vi "cos_rise_512_steps.vi"(9 "new step":bool, 10 "input valid":bool=TRUE, 11 "data in":fxp<+/-,16,1>) -> (1 "output valid":bool, 2 "steping":bool, 3 "data out":fxp<+/-,16,1>)   [LabVIEW 2021]
doc: "rise function.\n32 steps of half cos."
uses:
  <instrlib>/_niInstr/Basic Elements/v1/FPGA/Private/Count Up U16.vi
  <vilib>/rvi/FXPMathLib/FxpSub/XNode/nifxpmath_Sub.xnode
  <vilib>/rvi/FXPMathLib/FxpMul/XNode/nifxpmath_Multiplier.xnode
  <vilib>/rvi/FXPMathLib/FxpAdd/XNode/nifxpmath_Add.xnode
  <instrlib>/_niInstr/Basic Elements/v1/FPGA/niInstr Basic Elements v1 FPGA.lvlib
  <vilib>/rvi/FXPMathLib/sim/FxpSim.dll
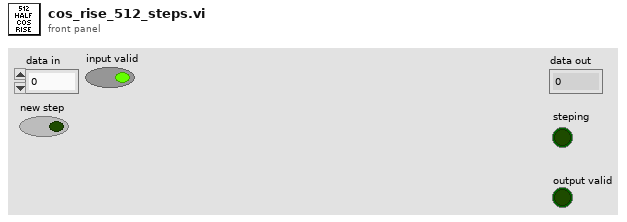
[diagram p1: front panel]
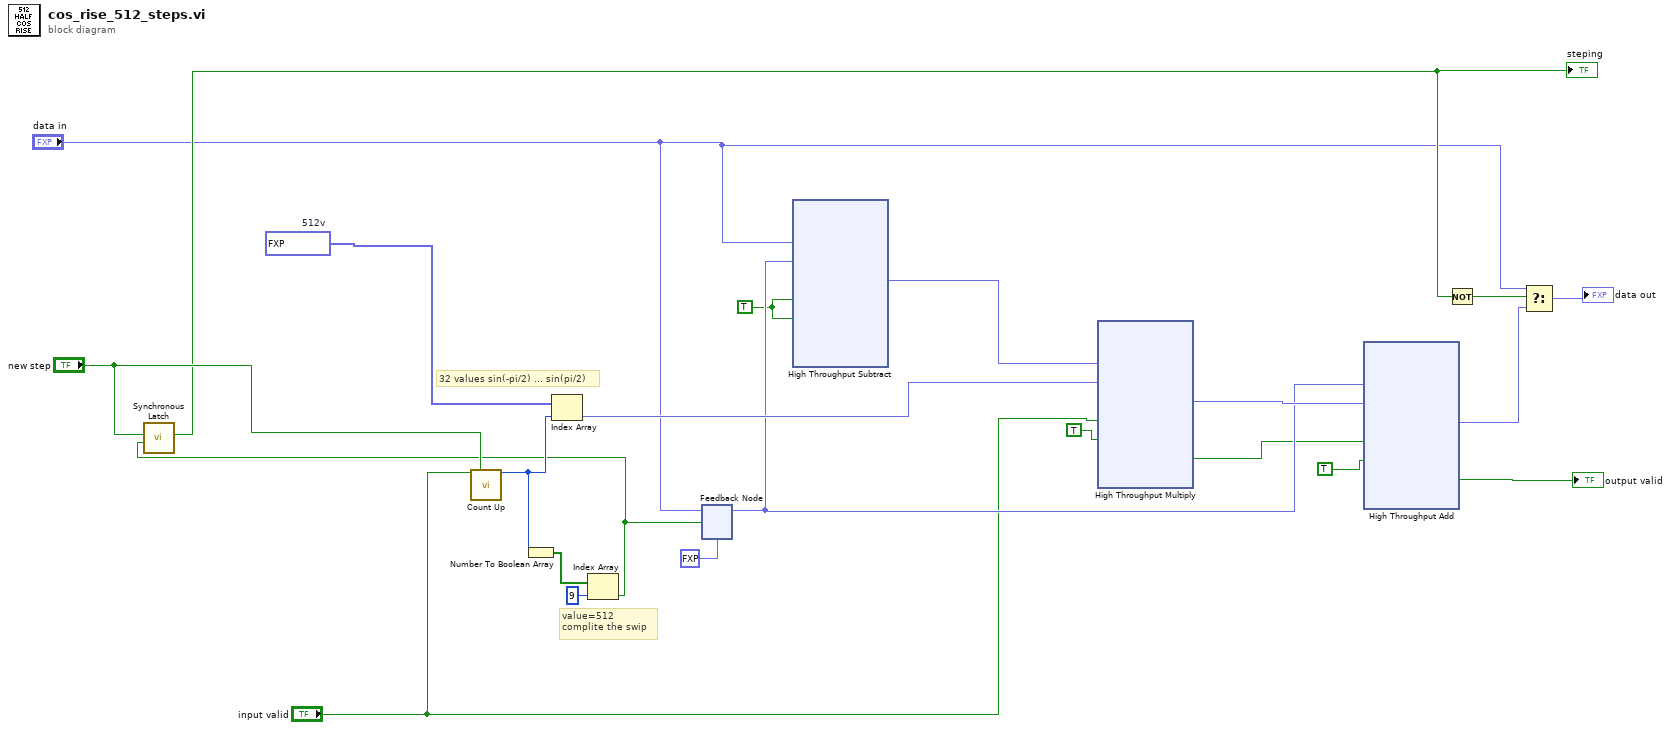
[diagram p0: block diagram]
diagram:
  w5 = fxp<+,24,0>[] [9.417533874511719e-06, 3.7670135498046875e-05, 8.469820022583008e-05, 0.00015056133270263672, 0.0002353191375732422, 0.0003387928009033203, 0.00046116113662719727, 0.0006022453308105469, 0.0007622241973876953, 0.0009409189224243164, 0.001138448715209961, 0.0013547539710998535, 0.0015898346900939941, 0.0018436908721923828, 0.0021163225173950195, 0.0024076104164123535, 0.002717733383178711, 0.0030465126037597656, 0.003394007682800293, 0.003760218620300293, 0.004145145416259766, 0.00454866886138916, 0.004970908164978027, 0.005411744117736816, 0.005871236324310303, 0.0063492655754089355, 0.006845951080322266, 0.007361173629760742, 0.007894933223724365, 0.008447229862213135, 0.00901806354522705, 0.009607374668121338, 0.01021510362625122, 0.010841310024261475, 0.011485934257507324, 0.012148916721343994, 0.01283031702041626, 0.01353001594543457, 0.014248073101043701, 0.014984369277954102, 0.015738964080810547, 0.016511738300323486, 0.017302751541137695, 0.0181119441986084, 0.018939316272735596, 0.019784748554229736, 0.02064824104309082, 0.021529853343963623, 0.02242940664291382, 0.02334696054458618, 0.024282515048980713, 0.025235891342163086, 0.02620720863342285, 0.02719634771347046, 0.028203248977661133, 0.02922797203063965, 0.030270397663116455, 0.03133046627044678, 0.03240823745727539, 0.033503592014312744, 0.03461652994155884, 0.03574693202972412, 0.03689485788345337, 0.03806024789810181, 0.03924298286437988, 0.0404430627822876, 0.04166048765182495, 0.04289513826370239, 0.044146955013275146, 0.04541599750518799, 0.04670214653015137, 0.04800534248352051, 0.04932558536529541, 0.05066275596618652, 0.05201685428619385, 0.05338782072067261, 0.0547756552696228, 0.05618017911911011, 0.0576014518737793, 0.05903935432434082, 0.06049388647079468, 0.06196492910385132, 0.06345248222351074, 0.06495648622512817, 0.06647688150405884, 0.06801354885101318, 0.06956654787063599, 0.07113569974899292, 0.07272100448608398, 0.0743224024772644, 0.0759398341178894, 0.07757323980331421, 0.07922250032424927, 0.08088767528533936, 0.08256858587265015, 0.08426517248153687, 0.08597749471664429, 0.08770537376403809, 0.08944875001907349, 0.09120756387710571, 0.09298181533813477, 0.0947713851928711, 0.09657621383666992, 0.09839624166488647, 0.1002313494682312, 0.1020815372467041, 0.10394668579101562, 0.10582679510116577, 0.10772168636322021, 0.10963135957717896, 0.11155575513839722, 0.11349475383758545, 0.11544835567474365, 0.1174163818359375, 0.11939883232116699, 0.12139558792114258, 0.12340658903121948, 0.12543177604675293, 0.12747108936309814, 0.12952440977096558, 0.13159173727035522, 0.13367289304733276, 0.13576781749725342, 0.1378764510154724, 0.13999873399734497, 0.14213460683822632, 0.14428389072418213, 0.1464465856552124, 0.14862263202667236, 0.15081185102462769, 0.15301424264907837, 0.15522974729537964, 0.15745818614959717, 0.15969949960708618, 0.1619536280632019, 0.16422051191329956, 0.1665000319480896, 0.16879212856292725, 0.17109668254852295, 0.17341357469558716, 0.17574280500411987, 0.17808425426483154, 0.18043780326843262, 0.18280333280563354, 0.1851809024810791, 0.18757027387619019, 0.18997138738632202, 0.19238418340682983, 0.19480860233306885, 0.19724446535110474, 0.1996917724609375, 0.2021503448486328, 0.2046201229095459, 0.20710104703903198, 0.2095929980278015, 0.21209591627120972, 0.21460962295532227, 0.21713411808013916, 0.21966922283172607, 0.22221487760543823, 0.22477102279663086, 0.22733747959136963, 0.22991424798965454, 0.23250120878219604, 0.23509818315505981, 0.23770517110824585, 0.24032199382781982, 0.24294865131378174, 0.2455849051475525, 0.24823081493377686, 0.25088614225387573, 0.2535508871078491, 0.25622493028640747, 0.25890809297561646, 0.2616003751754761, 0.2643016576766968, 0.26701176166534424, 0.2697306275367737, 0.27245819568634033, 0.27519434690475464, 0.2779389023780823, 0.28069186210632324, 0.283453106880188, 0.2862224578857422, 0.28899985551834106, 0.29178524017333984, 0.2945784330368042, 0.2973793148994446, 0.300187885761261, 0.3030039668083191, 0.3058274984359741, 0.30865830183029175, 0.3114963173866272, 0.3143414258956909, 0.31719350814819336, 0.32005250453948975, 0.32291823625564575, 0.3257906436920166, 0.3286696672439575, 0.3315550684928894, 0.33444684743881226, 0.33734482526779175, 0.3402490019798279, 0.34315913915634155, 0.346075177192688, 0.34899699687957764, 0.3519245386123657, 0.3548576831817627, 0.35779625177383423, 0.36074018478393555, 0.3636893033981323, 0.36664360761642456, 0.36960291862487793, 0.37256717681884766, 0.3755362033843994, 0.3785099387168884, 0.38148820400238037, 0.38447093963623047, 0.38745802640914917, 0.3904494047164917, 0.39344483613967896, 0.39644432067871094, 0.3994476795196533, 0.40245485305786133, 0.40546566247940063, 0.40848004817962646, 0.41149789094924927, 0.4145190715789795, 0.4175434112548828, 0.42057090997695923, 0.4236013889312744, 0.4266347885131836, 0.42967087030410767, 0.43270963430404663, 0.43575096130371094, 0.43879467248916626, 0.4418407082557678, 0.4448888897895813, 0.4479391574859619, 0.4509914517402649, 0.45404553413391113, 0.45710134506225586, 0.4601587653160095, 0.46321773529052734, 0.4662780165672302, 0.46933960914611816, 0.4724023938179016, 0.47546619176864624, 0.4785308837890625, 0.4815964102745056, 0.48466259241104126, 0.48772937059402466, 0.49079662561416626, 0.4938642382621765, 0.4969320297241211, 0.5, 0.5030679702758789, 0.5061357617378235, 0.5092033743858337, 0.5122706294059753, 0.5153374075889587, 0.5184035897254944, 0.5214691162109375, 0.5245338082313538, 0.5275976061820984, 0.5306603908538818, 0.5337219834327698, 0.5367822647094727, 0.5398412346839905, 0.5428986549377441, 0.5459544658660889, 0.5490085482597351, 0.5520608425140381, 0.5551111102104187, 0.5581592917442322, 0.5612053275108337, 0.5642490386962891, 0.5672903656959534, 0.5703291296958923, 0.5733652114868164, 0.5763986110687256, 0.5794290900230408, 0.5824565887451172, 0.5854809284210205, 0.5885021090507507, 0.5915199518203735, 0.5945343375205994, 0.5975451469421387, 0.6005523204803467, 0.6035556793212891, 0.606555163860321, 0.6095505952835083, 0.6125419735908508, 0.6155290603637695, 0.6185117959976196, 0.6214900612831116, 0.6244637966156006, 0.6274328231811523, 0.6303970813751221, 0.6333563923835754, 0.6363106966018677, 0.6392598152160645, 0.6422037482261658, 0.6451423168182373, 0.6480754613876343, 0.6510030031204224, 0.653924822807312, 0.6568408608436584, 0.6597509980201721, 0.6626551747322083, 0.6655531525611877, 0.6684449315071106, 0.6713303327560425, 0.6742093563079834, 0.6770817637443542, 0.6799474954605103, 0.6828064918518066, 0.6856585741043091, 0.6885036826133728, 0.6913416981697083, 0.6941725015640259, 0.6969960331916809, 0.699812114238739, 0.7026206851005554, 0.7054215669631958, 0.7082147598266602, 0.7110001444816589, 0.7137775421142578, 0.716546893119812, 0.7193081378936768, 0.7220610976219177, 0.7248056530952454, 0.7275418043136597, 0.7302693724632263, 0.7329882383346558, 0.7356983423233032, 0.7383996248245239, 0.7410919070243835, 0.7437750697135925, 0.7464491128921509, 0.7491138577461243, 0.7517691850662231, 0.7544150948524475, 0.7570513486862183, 0.7596780061721802, 0.7622948288917542, 0.7649018168449402, 0.767498791217804, 0.7700857520103455, 0.7726625204086304, 0.7752289772033691, 0.7777851223945618, 0.7803307771682739, 0.7828658819198608, 0.7853903770446777, 0.7879040837287903, 0.7904070019721985, 0.792898952960968, 0.7953798770904541, 0.7978496551513672, 0.8003082275390625, 0.8027555346488953, 0.8051913976669312, 0.8076158165931702, 0.810028612613678, 0.8124297261238098, 0.8148190975189209, 0.8171966671943665, 0.8195621967315674, 0.8219157457351685, 0.8242571949958801, 0.8265864253044128, 0.828903317451477, 0.8312078714370728, 0.8334999680519104, 0.8357794880867004, 0.8380463719367981, 0.8403005003929138, 0.8425418138504028, 0.8447702527046204, 0.8469857573509216, 0.8491881489753723, 0.8513773679733276, 0.8535534143447876, 0.8557161092758179, 0.8578653931617737, 0.860001266002655, 0.8621235489845276, 0.8642321825027466, 0.8663271069526672, 0.8684082627296448, 0.8704755902290344, 0.8725289106369019, 0.8745682239532471, 0.8765934109687805, 0.8786044120788574, 0.880601167678833, 0.8825836181640625, 0.8845516443252563, 0.8865052461624146, 0.8884442448616028, 0.890368640422821, 0.8922783136367798, 0.8941732048988342, 0.8960533142089844, 0.8979184627532959, 0.8997686505317688, 0.9016037583351135, 0.9034237861633301, 0.9052286148071289, 0.9070181846618652, 0.9087924361228943, 0.9105512499809265, 0.9122946262359619, 0.9140225052833557, 0.9157348275184631, 0.9174314141273499, 0.9191123247146606, 0.9207774996757507, 0.9224267601966858, 0.9240601658821106, 0.9256775975227356, 0.927278995513916, 0.9288643002510071, 0.930433452129364, 0.9319864511489868, 0.9335231184959412, 0.9350435137748718, 0.9365475177764893, 0.9380350708961487, 0.9395061135292053, 0.9409606456756592, 0.9423985481262207, 0.9438198208808899, 0.9452243447303772, 0.9466121792793274, 0.9479831457138062, 0.9493372440338135, 0.9506744146347046, 0.9519946575164795, 0.9532978534698486, 0.954584002494812, 0.9558530449867249, 0.9571048617362976, 0.958339512348175, 0.9595569372177124, 0.9607570171356201, 0.9619397521018982, 0.9631051421165466, 0.9642530679702759, 0.9653834700584412, 0.9664964079856873, 0.9675917625427246, 0.9686695337295532, 0.9697296023368835, 0.9707720279693604, 0.9717967510223389, 0.9728036522865295, 0.9737927913665771, 0.9747641086578369, 0.9757174849510193, 0.9766530394554138, 0.9775705933570862, 0.9784701466560364, 0.9793517589569092, 0.9802152514457703, 0.9810606837272644, 0.9818880558013916, 0.9826972484588623, 0.9834882616996765, 0.9842610359191895, 0.9850156307220459, 0.9857519268989563, 0.9864699840545654, 0.9871696829795837, 0.987851083278656, 0.9885140657424927, 0.9891586899757385, 0.9897848963737488, 0.9903926253318787, 0.990981936454773, 0.9915527701377869, 0.9921050667762756, 0.9926388263702393, 0.9931540489196777, 0.9936507344245911, 0.9941287636756897, 0.9945882558822632, 0.995029091835022, 0.9954513311386108, 0.9958548545837402, 0.9962397813796997, 0.9966059923171997, 0.9969534873962402, 0.9972822666168213, 0.9975923895835876, 0.997883677482605, 0.9981563091278076, 0.998410165309906, 0.9986452460289001, 0.99886155128479, 0.9990590810775757, 0.9992377758026123, 0.9993977546691895, 0.9995388388633728, 0.9996612071990967, 0.9997646808624268, 0.9998494386672974, 0.9999153017997742, 0.999962329864502, 0.9999905824661255, 0.9999999403953552]  # 512v
  w4 = TRUE ("input valid")
  # "value=512\ncomplite the swip"
  # "32 values sin(-pi/2) ... sin(pi/2)"
  n1 = call-poly <instrlib>:"Count Up.vi"("increment"="input valid", "reset"="new step") -> ("count out"=w15:u16)  [unwired: 13 in]
  n2 = Number To Boolean Array(number=w15) -> (Boolean array=w14:bool[])
  n3 = Index Array(array=w5, index=w15) -> (element=w22:fxp<+,24,0>)
  n4 = Index Array(array=w14, index=9) -> (element=w12:bool)
  n5 = call <instrlib>:"Synchronous Latch.vi"("clear"=w12, "set"="new step") -> ("out"=w10:bool)  [unwired: 9 in]
  "steping" <- w10
  n6 = feedback-in #1("data in", w12) -> ()
  n7 = feedback #1(fxp<+/-,16,1> 0.0 ("data in")) -> (w6:fxp<+/-,16,1>)
  n8 = xnode "High Throughput Subtract"("x"="data in", "y"=w6, "input valid"=w4, "ready for output (T)"=w4) -> ("x-y"=w19:fxp<+/-,16,1>)  [unwired: 2 out]
  n9 = xnode ("High Throughput Multiply")("x"=w19, "y"=w22, "input valid"="input valid", "ready for output (T)"=TRUE ("input valid")) -> ("x*y"=w20:fxp<+/-,16,1>, "output valid"=w2:bool)  [unwired: 1 out]
  n10 = xnode ("High Throughput Add")("x"=w6, "y"=w20, "input valid"=w2, "ready for output (T)"=TRUE ("input valid")) -> ("x+y"=w18:fxp<+/-,16,1>, "output valid"=→"output valid":bool)  [unwired: 1 out]
  n11 = Not(x=w10) -> (.not. x?=w11:bool)
  n12 = Select(t="data in", s=w11, f=w18) -> (s? t:f=→"data out":fxp<+/-,16,1>)
